vi "Preview Input Channel.vi"(7 "channel":i32, 8 "error in":errorcluster, 10 "samples":u32=2048, 11 "fpga session in":refnum<k20>) -> (0 "error out":errorcluster, 2 "ai data":i16[](array[numeric]), 3 "fpga session out":refnum<k20>)   [LabVIEW 2017, in "Lock-In Amplifier Example Host.lvlib"]
uses:
  Lock-In Amplifier Example Host.lvlib
  fpga type.ctl
  <vilib>/Utility/error.llb/Error Cluster From Error Code.vi
  <vilib>/rvi/errors/niLvFpgaAdjustHostInterfaceError.vi
  <instrlib>/_niInstr/Streaming/v1/Host/Public/Start Finite Stream.vi
  <vilib>/rvi/interface/nirviReadWriteControl/nirviReadWriteControl.xnode
  <vilib>/rvi/interface/nirviMethod/nirviMethod.xnode
  <instrlib>/_niInstr/Streaming/v1/Host/niInstr Streaming v1 Host.lvlib
  NiFpgaLv.dll
  <vilib>/rvi/interface/Simulation/niFpgaSimulationCallBeginRW.vi
  <vilib>/FPGAPlugInAG/Dynamic/niLvFpga_ReadFifo_Dynamic.vi
  <vilib>/rvi/errors/niLvFpgaMergeErrorWithErrorCode.vi
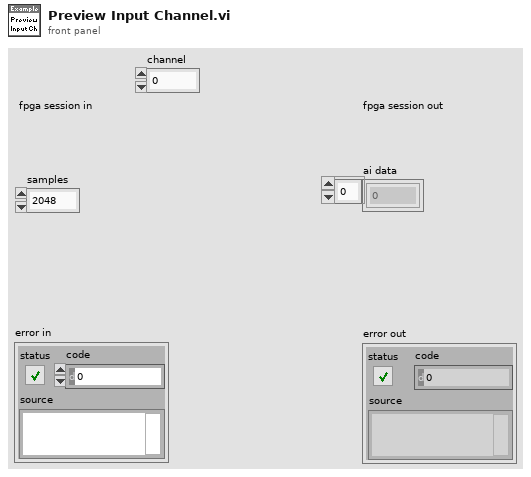
[diagram p1: front panel]
types:
  T1 = typedef "Lock-In Amplifier Example Host.lvlib/fpga type.ctl" = refnum<k20>
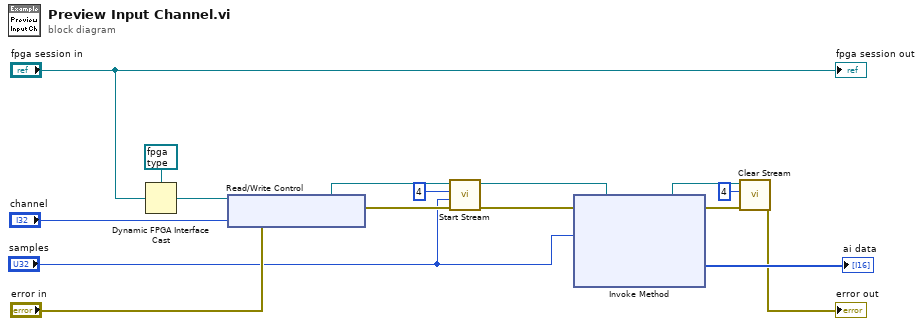
[diagram p0: block diagram]
diagram:
  n1 = Dynamic FPGA Interface Cast(Session In=T1 refnum ("fpga type"), Type="fpga session in") -> (Session Out=w14:T1)
  n2 = xnode "Read/Write Control"("FPGA VI Reference In"=w14, "error in"="error in", "preview.channel select"="channel") -> ("FPGA VI Reference Out"=w10:T1, "error out"=w11:errorcluster)
  n3 = call-poly <instrlib>:"Start Stream.vi"("error in (no error)"=w11, "num samples"="samples", "stream index"=4, "refnum in"=w10) -> ("error out"=w7:errorcluster, "refnum out"=w8:T1)  [unwired: 6 in]
  n4 = xnode "Invoke Method"("FPGA VI Reference In"=w8, "error in"=w7, "Number of Elements"="samples") -> ("FPGA VI Reference Out"=w4:T1, "error out"=w3:errorcluster, "Data"=→"ai data":i16[])  [unwired: 1 in, 1 out]
  n5 = call <instrlib>:"Clear Stream.vi"("error in (no error)"=w3, "stream index"=4, "refnum in"=w4) -> ("error out"=→"error out":errorcluster)  [unwired: 7 in, 1 out]
  "fpga session out" <- "fpga session in"
